vi "flot graph.vi"(7 "BD Date":string[](array[string]), 8 "error in (no error)":errorcluster) -> (3 "Run-Time Status":cluster{"Array 2":timestamp[], dbl[]}(graph))   [LabVIEW 2017]
panel:
  out "element":timestamp
  out "Elements Found out 2":string[](array[string])
  out "Count out 2":string[](array[string])
  in  "1":dbl format="%#_13g"
  out "XY Graph":cluster{"Array 2":timestamp[], dbl[]}(graph)
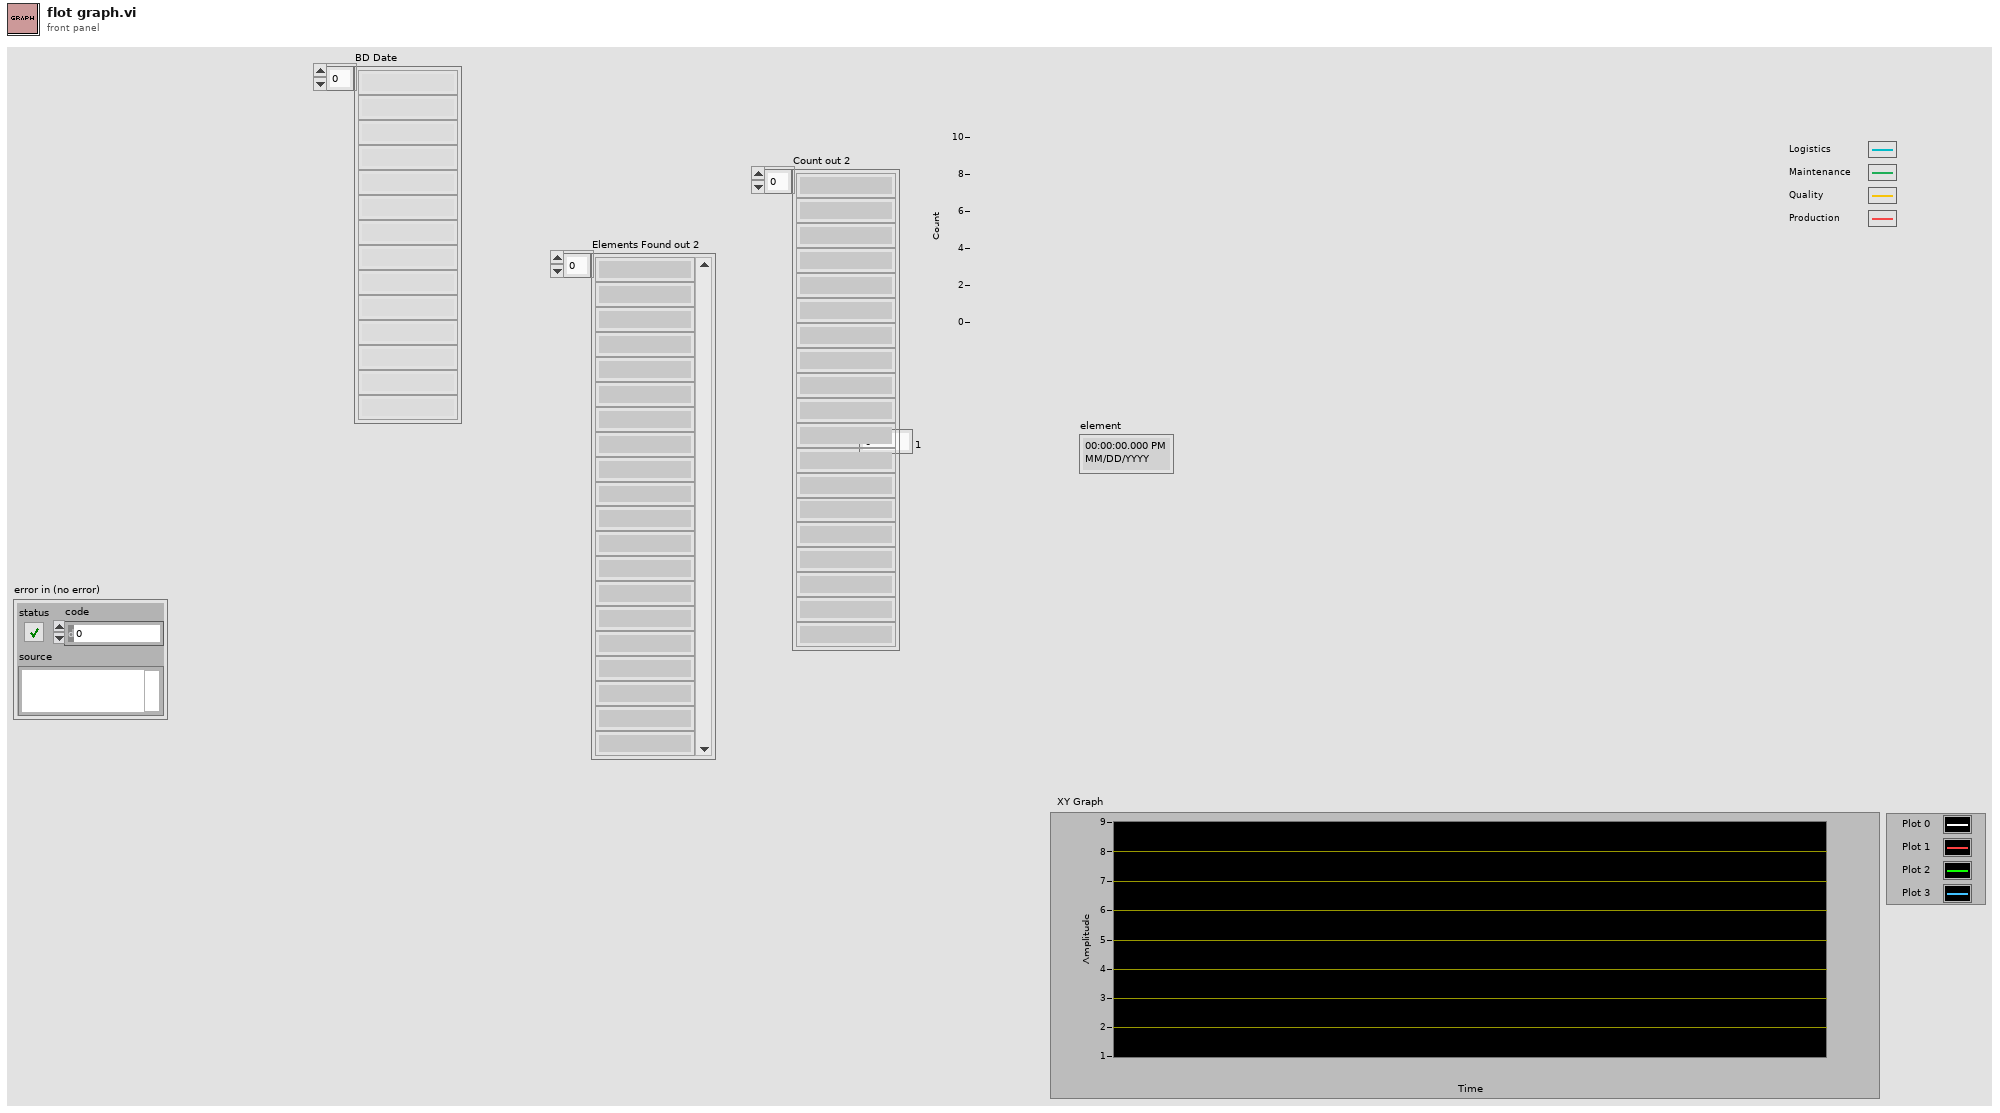
[diagram p1: front panel]
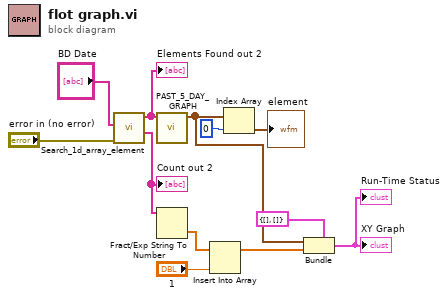
[diagram p0: block diagram]
diagram:
  n1 = call "Search_1d_array_element.vi"("error in (no error)"="error in (no error)", "BD Date"="BD Date") -> ("Count out"=w3:string[], "Elements Found out"=w4:string[])  [unwired: 5 in, 1 out]
  "Count out 2" <- w3
  "Elements Found out 2" <- w4
  n2 = call "PAST_5_DAY_GRAPH.vi"("5 date"=w4) -> ("Array 2"=w8:timestamp[])  [unwired: 9 in, 1 out]
  n3 = Fract/Exp String To Number(string=w3) -> (number=w11:dbl[])  [unwired: 3 in, 1 out]
  n4 = Insert Into Array(array=w11, new element="1") -> (w10:dbl[])  [unwired: 1 in]
  n5 = Index Array(array=w8, index=0) -> (element=→"element":timestamp)
  n6 = Bundle(cluster=cluster{"Array 2":timestamp[], dbl[]} {"Array 2"=[], []}, "Array 2"=w8, w10) -> (→"XY Graph" →"Run-Time Status":cluster{"Array 2":timestamp[], dbl[]})
